vi "Module Loop.vi"(8 "error in (no error)":errorcluster, 11 "Redlines Module in":refnum<class "Redlines Module.lvclass">) -> (0 "error out":errorcluster, 3 "Redlines Module out":refnum<class "Redlines Module.lvclass">)   [LabVIEW 2020, in "VolatusData.lvlib" / "Redlines Module.lvclass"]
uses:
  Redlines Module.lvclass
  Redlines Module.lvclass/Redlines Module.ctl
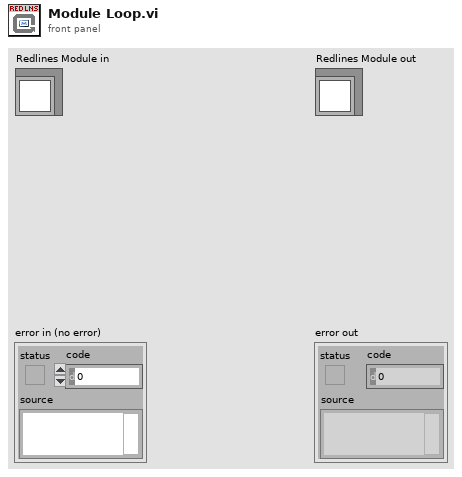
[diagram p1: front panel]
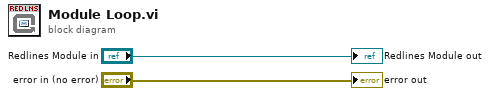
[diagram p0: block diagram]
diagram:
  "error out" <- "error in (no error)"
  "Redlines Module out" <- "Redlines Module in"
